vi "Custom_Create_VI_Documentation_Component_Image.vi"(6 "special chars in file path of image":string, 7 "Content Options":T1, 8 "error in (no error)":errorcluster, 9 "Image Depth":i32=24, 10 "Image Format (jpeg)":enum32{"PNG", "JPEG", "GIF"}(ring)=enum."JPEG", 11 "VI":refnum<vi>) -> (0 "error out":errorcluster, 3 "Path to image":path)   [LabVIEW 2019]
uses:
  <vilib>/printing/ReportDocExtensions.llb/File_types_for_reports.ctl
  <vilib>/Utility/NIReport.llb/NI_ReportGenerationCore.lvlib
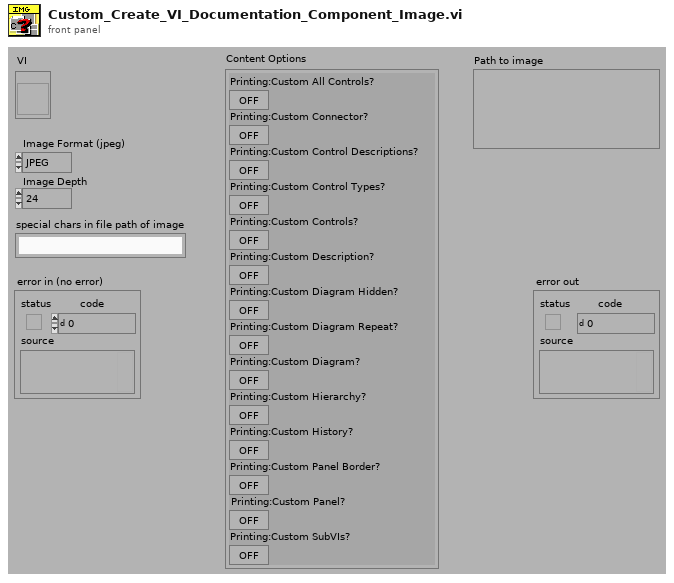
[diagram p1: front panel]
types:
  T1 = cluster{"Printing:Custom All Controls?":bool, "Printing:Custom Connector?":bool, "Printing:Custom Control Descriptions?":bool, "Printing:Custom Control Types?":bool, "Printing:Custom Controls?":bool, "Printing:Custom Description?":bool, "Printing:Custom Diagram Hidden?":bool, "Printing:Custom Diagram Repeat?":bool, "Printing:Custom Diagram?":bool, "Printing:Custom Hierarchy?":bool, "Printing:Custom History?":bool, "Printing:Custom Panel Border?":bool, "Printing:Custom Panel?":bool, "Printing:Custom SubVIs?":bool}
  T2 = typedef "NI_ReportGenerationCore.lvlib/File_types_for_reports.ctl" = enum16{".jpg", ".png", ".html", ".gif"}
  T3 = enum32{"Custom", "Standard", "Using Panel", "Using SubVI", "Complete"}
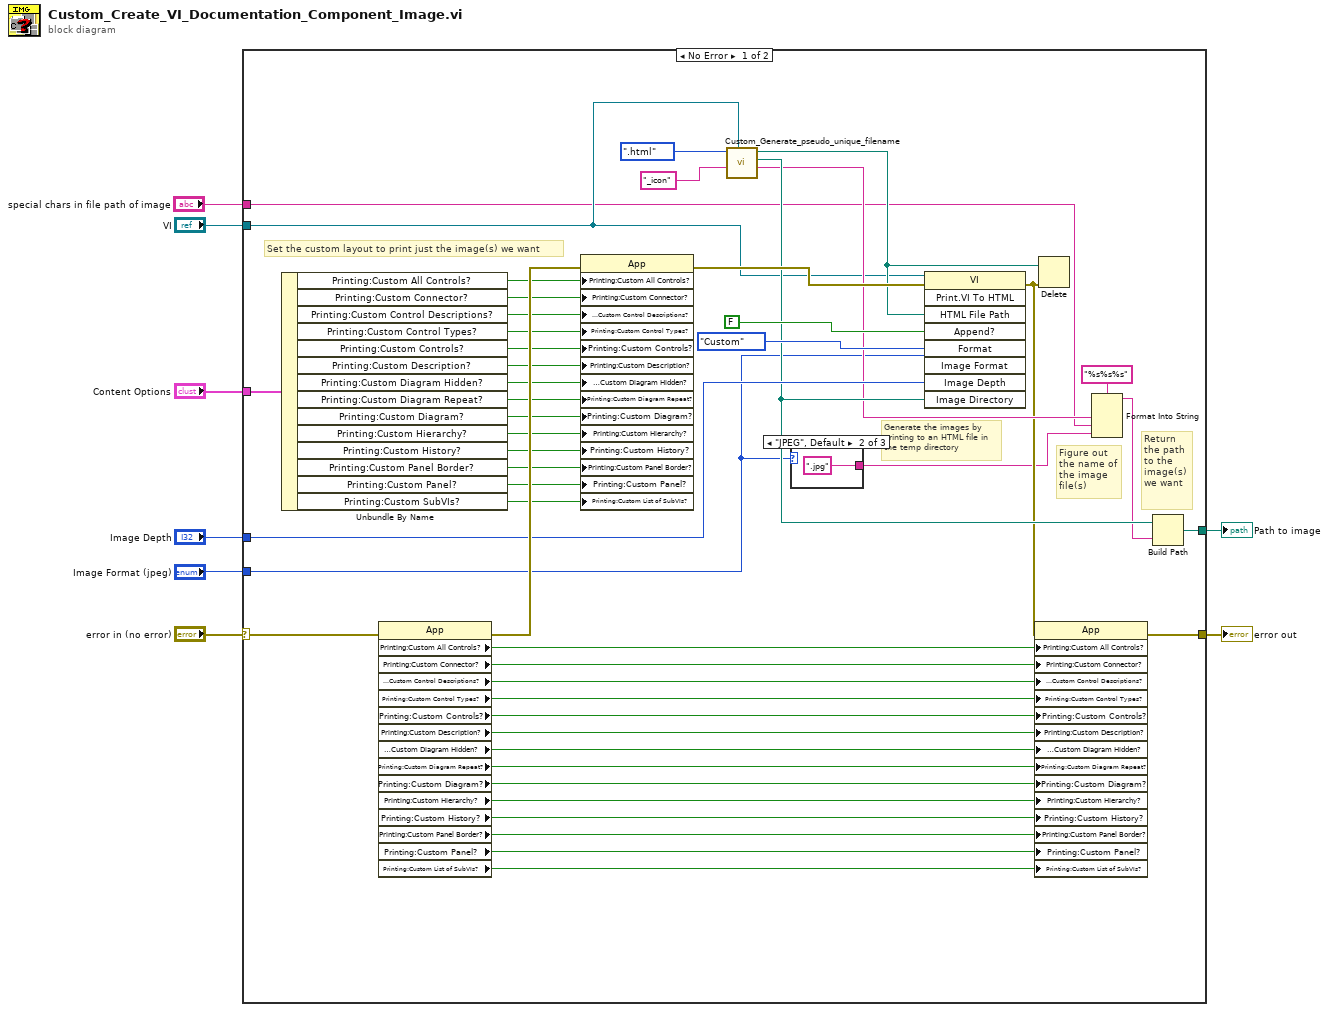
[diagram p0: block diagram]
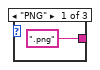
[diagram p2: hidden frame]
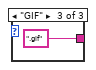
[diagram p3: hidden frame]
diagram:
  n1 = case shown="No Error" "error in (no error)" {
    selector: "error in (no error)" -> [w14 w61]
    tunnel: [w43 w61] -> w8
    tunnel: "VI" -> [w12 _]
    tunnel: "Image Depth" -> [w40 _]
    tunnel: [w33 _] -> w5
    tunnel: "Content Options" -> [w31 _]
    tunnel: "special chars in file path of image" -> [w9 _]
    tunnel: "Image Format (jpeg)" -> [w16 _]
    frame No Error {
      # "Figure out the name of the image file(s)"
      # "Return the path to the image(s) we want"
      # "Generate the images by printing to an HTML file in the temp directory"
      # "Set the custom layout to print just the image(s) we want"
      n2 = Unbundle By Name(w31) -> ("Printing:Custom All Controls?"=w30:bool, "Printing:Custom Connector?"=w29:bool, "Printing:Custom Control Descriptions?"=w28:bool, "Printing:Custom Control Types?"=w27:bool, "Printing:Custom Controls?"=w26:bool, "Printing:Custom Description?"=w25:bool, "Printing:Custom Diagram Hidden?"=w24:bool, "Printing:Custom Diagram Repeat?"=w23:bool, "Printing:Custom Diagram?"=w22:bool, "Printing:Custom Hierarchy?"=w21:bool, "Printing:Custom History?"=w20:bool, "Printing:Custom Panel Border?"=w19:bool, "Printing:Custom Panel?"=w18:bool, "Printing:Custom SubVIs?"=w17:bool)
      n3 = property class="App"(error in=w14) -> (error out=w42:errorcluster, "Printing:Custom All Controls?"=w44:bool, "Printing:Custom Connector?"=w45:bool, "Printing:Custom Control Descriptions?"=w46:bool, "Printing:Custom Control Types?"=w47:bool, "Printing:Custom Controls?"=w48:bool, "Printing:Custom Description?"=w49:bool, "Printing:Custom Diagram Hidden?"=w50:bool, "Printing:Custom Diagram Repeat?"=w51:bool, "Printing:Custom Diagram?"=w52:bool, "Printing:Custom Hierarchy?"=w53:bool, "Printing:Custom History?"=w54:bool, "Printing:Custom Panel Border?"=w55:bool, "Printing:Custom Panel?"=w56:bool, "Printing:Custom List of SubVIs?"=w57:bool)  [unwired: 1 in, 1 out]
      n4 = property class="App"(error in=w42, "Printing:Custom All Controls?"=w30, "Printing:Custom Connector?"=w29, "Printing:Custom Control Descriptions?"=w28, "Printing:Custom Control Types?"=w27, "Printing:Custom Controls?"=w26, "Printing:Custom Description?"=w25, "Printing:Custom Diagram Hidden?"=w24, "Printing:Custom Diagram Repeat?"=w23, "Printing:Custom Diagram?"=w22, "Printing:Custom Hierarchy?"=w21, "Printing:Custom History?"=w20, "Printing:Custom Panel Border?"=w19, "Printing:Custom Panel?"=w18, "Printing:Custom List of SubVIs?"=w17) -> (error out=w41:errorcluster)  [unwired: 1 in, 1 out]
      n5 = call "Custom_Generate_pseudo_unique_filename.vi"("VI"=w12, "Suffix"="_icon", "file type(.jpg)"=File_types_for_reports.".html") -> ("root filename"=w32:string, "temp directory"=w35:path, "generated path"=w13:path)  [unwired: 6 in]
      n6 = case shown="\"JPEG\", Default" w16 {
        tunnel: [".png" ".jpg" ".gif"] -> w10
        frame "PNG" {
        }
        frame "JPEG", Default {
        }
        frame "GIF" {
        }
      }
      n7 = invoke class="VI" method="Print.VI To HTML"(reference=w12, error in=w41, "HTML File Path"=w13, "Append?"=FALSE, "Format"=T3."Custom", "Image Format"=w16, "Image Depth"=w40, "Image Directory"=w35) -> (error out=w15:errorcluster)  [unwired: 1 in, 8 out]
      n8 = property class="App"(error in=w15, "Printing:Custom All Controls?"=w44, "Printing:Custom Connector?"=w45, "Printing:Custom Control Descriptions?"=w46, "Printing:Custom Control Types?"=w47, "Printing:Custom Controls?"=w48, "Printing:Custom Description?"=w49, "Printing:Custom Diagram Hidden?"=w50, "Printing:Custom Diagram Repeat?"=w51, "Printing:Custom Diagram?"=w52, "Printing:Custom Hierarchy?"=w53, "Printing:Custom History?"=w54, "Printing:Custom Panel Border?"=w55, "Printing:Custom Panel?"=w56, "Printing:Custom List of SubVIs?"=w57) -> (error out=w43:errorcluster)  [unwired: 1 in, 1 out]
      n9 = Delete(path (use dialog)=w13, error in=w15) -> ()  [unwired: 3 in, 3 out]
      n10 = Format Into String(format string="%s%s%s" ("Format String"), w32, w9, w10) -> (resulting string=w34:string)  [unwired: 2 in, 1 out]
      n11 = Build Path(base path=w35, name or relative path=w34) -> (appended path=w33:path)
    }
    frame Error {
    }
  }
  "error out" <- w8
  "Path to image" <- w5
